vi "QTMTest.vi"() -> ()   [LabVIEW 2014]
uses:
  CustomIO.ctl
  Oqus Custom Device.lvlib
panel:
  out "return count":u32
  in  "timeout ms (25000)":i32=6000
  out "Waveform Chart":dbl(graph)
  in  "SamplingRate [ms]":u32
  in  "stop":bool
  out "error out":errorcluster
  out "DataOut":dbl[](array[numeric])
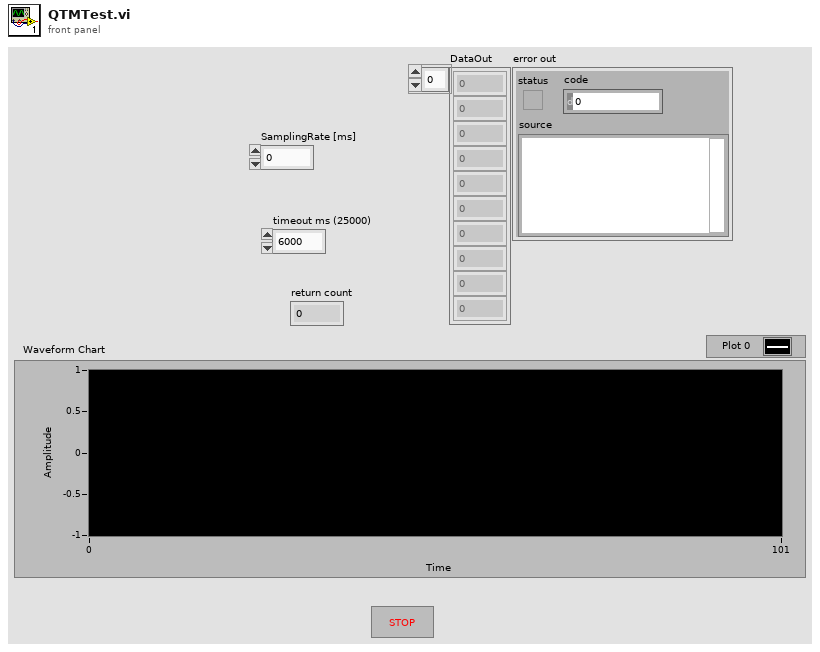
[diagram p1: front panel]
types:
  T1 = typedef "Oqus Custom Device.lvlib/CustomIO.ctl" = enum16{"Init", "Read", "Write", "Close", "N/O"}
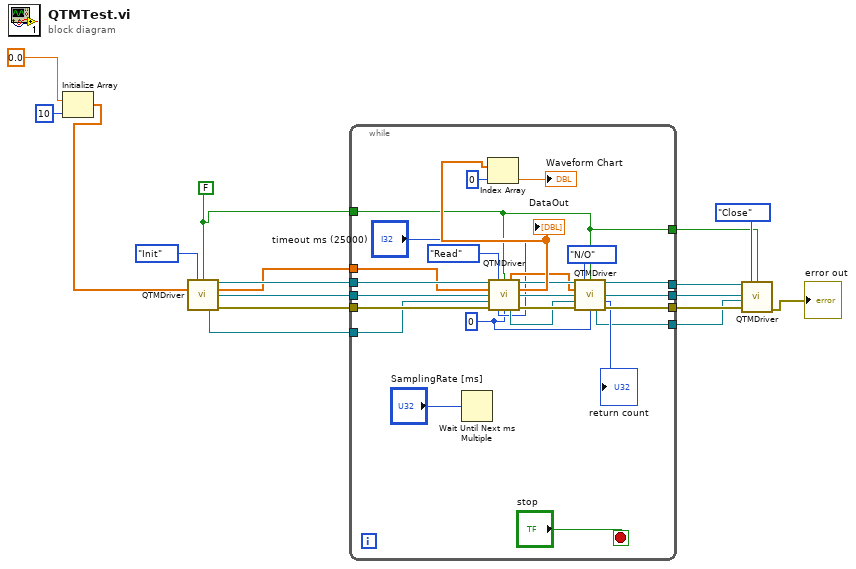
[diagram p0: block diagram]
diagram:
  w2 = FALSE ("WriteEnable")
  n1 = Initialize Array(0.0, 10 ("dimension size")) -> (w4:dbl[])
  n2 = call "QTMDriver.vi"("Ring"=CustomIO."Init", "WriteEnable"=w2, "DataIn"=w4) -> ("connection ID out"=w16:refnum<k5>, "DataOut"=w3:dbl[], "QTMqueue Out"=w8:refnum<queue>, "VI Refnum QTMTask Out"=w7:refnum<vi>, "error out"=w15:errorcluster)  [unwired: 6 in, 2 out]
  n3 = while {
    tunnel: w16 -> [w41]
    tunnel: w15 -> [w40]
    tunnel: w3 -> [w39]
    tunnel: [w29] -> w11
    tunnel: [w31] -> w10
    tunnel: w8 -> [w24]
    tunnel: w7 -> [w23]
    tunnel: [w22] -> w6
    tunnel: [w21] -> w5
    tunnel: w2 -> [w18]
    tunnel: [w18] -> w1
    stop <- "stop" stop-if-true
    w19 = 0 ("DataOutIndex")
    n4 = Wait Until Next ms Multiple(millisecond multiple="SamplingRate [ms]") -> ()  [unwired: 1 out]
    n5 = call "QTMDriver.vi"("connection ID"=w41, "Ring"=CustomIO."Read", "WriteEnable"=w18, "DataIn"=w39, "QTMqueue"=w24, "VI Refnum QTMTask"=w23, "error in"=w40, "timeout ms (25000)"="timeout ms (25000)", "DataOutIndex"=w19) -> ("ArrayOut"=w27:dbl[], "connection ID out"=w30:refnum<k5>, "DataOut"=w35:dbl[], "QTMqueue Out"=w26:refnum<queue>, "VI Refnum QTMTask Out"=w25:refnum<vi>, "error out"=w33:errorcluster)  [unwired: 1 out]
    "DataOut" <- w35
    n6 = Index Array(array=w35, index=0) -> (element=→"Waveform Chart":dbl)
    n7 = call "QTMDriver.vi"("connection ID"=w30, "Ring"=CustomIO."N/O", "WriteEnable"=w18, "DataIn"=w27, "QTMqueue"=w26, "VI Refnum QTMTask"=w25, "error in"=w33, "DataOutIndex"=w19) -> ("connection ID out"=w29:refnum<k5>, "QTMqueue Out"=w22:refnum<queue>, "return count"=→"return count":u32, "VI Refnum QTMTask Out"=w21:refnum<vi>, "error out"=w31:errorcluster)  [unwired: 1 in, 2 out]
  }
  n8 = call "QTMDriver.vi"("connection ID"=w11, "Ring"=CustomIO."Close", "WriteEnable"=w1, "QTMqueue"=w6, "VI Refnum QTMTask"=w5, "error in"=w10) -> ("error out"=→"error out":errorcluster)  [unwired: 3 in, 6 out]
